vi "Configure Continuous Acquisition.vi"(8 "error in (no error)":errorcluster, 10 "Enable Continuous Acquisition Mode (T:Enable)":bool=TRUE, 11 "VISA resource name":refnum<visa-resource-name>) -> (0 "error out":errorcluster, 3 "VISA resource name out":refnum<visa-resource-name>)   [LabVIEW 2015, in "Agilent 2000 3000 X-Series.lvlib"]
doc: "Configures the instrument to run continuously or to stop after a single configured acquisition.\n\n<B>Note(s):</B>\n(1) This setting does not occur until the Initiate VI or Read Waveform VI is called.\n(2) Performing an Autosetup puts the instrument in continuous acquisition mode."
uses:
  <instrlib>/Agilent 2000 3000 X-Series/Agilent 2000 3000 X-Series.lvlib
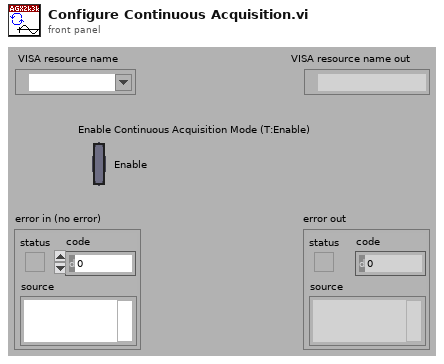
[diagram p1: front panel]
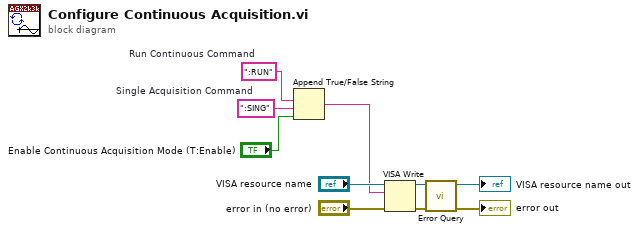
[diagram p0: block diagram]
diagram:
  w7 = ":SING"  # Single Acquisition Command
  w8 = ":RUN"  # Run Continuous Command
  n1 = Append True/False String(1:"Enable Continuous Acquisition Mode (T:Enable)", 2:w7, 3:w8) -> (0:w5:string)  [unwired: 1 out]
  n2 = VISA Write(VISA resource name="VISA resource name", write buffer=w5, error in (no error)="error in (no error)") -> (VISA resource name out=w4:refnum<visa-resource-name>, error out=w3:errorcluster)  [unwired: 1 out]
  n3 = call <instrlib>:"Error Query.vi"("error in (no error)"=w3, "VISA resource name"=w4) -> ("error out"=→"error out":errorcluster, "VISA resource name out"=→"VISA resource name out":refnum<visa-resource-name>)  [unwired: 8 out]
